vi "SelectOPCTags.AddItems.vi"(6 "VS Refs":T1[](array[typedef]) format="%.0x", 8 "error in (no error)":errorcluster, 9 "LUT":variant, 10 "Items":string[](array[string]), 11 "TreeControl in":refnum<vi>) -> (0 "error out":errorcluster)   [LabVIEW 2019, in "OPC UA Client Addon System Explorer.lvlib"]
uses:
  OPC UA Client Addon System Explorer.lvlib
  <vilib>/NI VeriStand/Custom Device API/Custom Device Item Ref.ctl
  Types/Tag.TreeSettings.ctl
  <vilib>/NI VeriStand/Custom Device API/Custom Device Channel.ctl
  <vilib>/NI VeriStand/Custom Device API/Custom Device Channel Type.ctl
  Addon Shared/Constants.vi
  <vilib>/NI VeriStand/Custom Device API/Set Item Property (U32).vi
  <vilib>/NI VeriStand/Custom Device API/Set Item Property (String).vi
  <vilib>/NI VeriStand/Custom Device API/Custom Device API.lvlib
  Addon Shared/OPC UA Client Addon Shared.lvlib
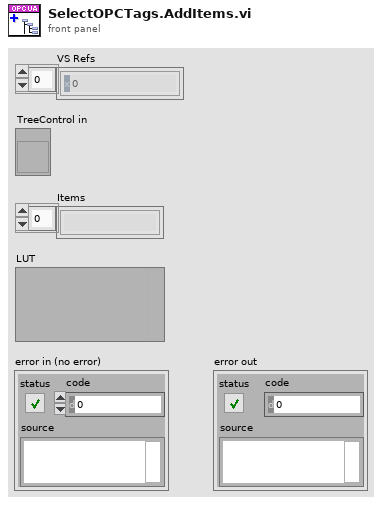
[diagram p1: front panel]
types:
  T1 = typedef "Custom Device API.lvlib/Custom Device Item Ref.ctl" = u64
  T2 = typedef "OPC UA Client Addon System Explorer.lvlib/Tag.TreeSettings.ctl" = cluster{"Settings":cluster{"name":string, "node type":enum32{"Other", "Folder", "Item/Property"}, "DataType":u32, "access":enum16{"Null", "Read", "Write", "Read&Write"}, "description":string}, "Array Size":i32}
  T3 = typedef "Custom Device API.lvlib/Custom Device Channel.ctl" = cluster{"Type":T4, "Units":string, "Default Value":dbl, "Faultable":bool, "Scalable":bool}
  T4 = typedef "Custom Device API.lvlib/Custom Device Channel Type.ctl" = enum16{"Input", "Output"}
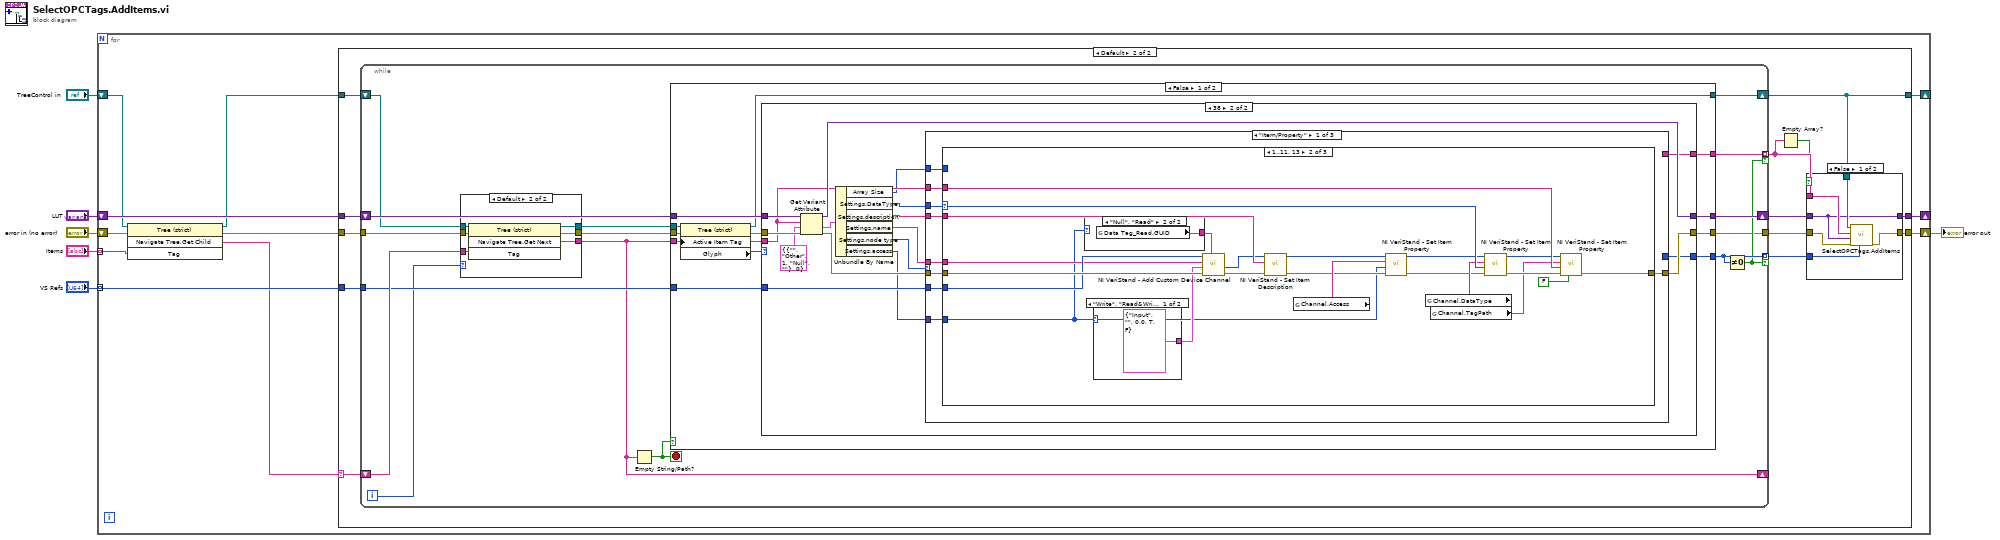
[diagram p0: block diagram]
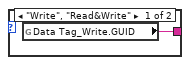
[diagram p7: hidden frame]
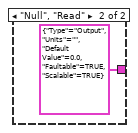
[diagram p8: hidden frame]
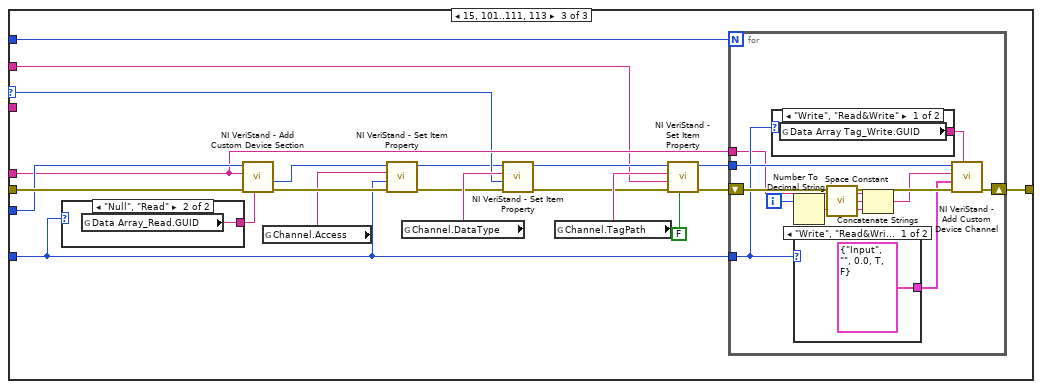
[diagram p9: hidden frame]
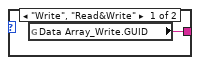
[diagram p10: hidden frame]
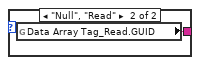
[diagram p11: hidden frame]
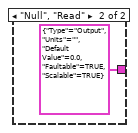
[diagram p12: hidden frame]
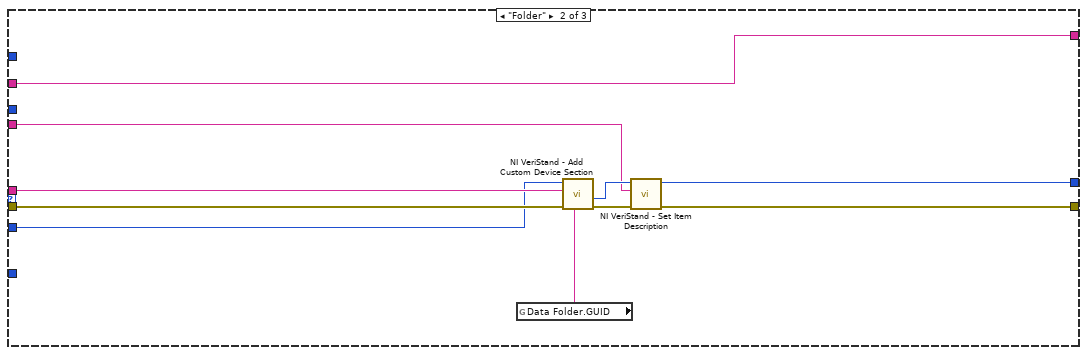
[diagram p13: hidden frame]
diagram:
  n1 = for {
    tunnel: "Items" -> [w8] mode=indexing
    tunnel: "VS Refs" -> [w17] mode=indexing
    shift-right: [w14] -> w1
    shift-left: "error in (no error)" -> [w12]
    shift-right: [w13] -> _
    shift-left: "LUT" -> [w16]
    shift-right: [w15] -> _
    shift-left: "TreeControl in" -> [w10]
    n2 = invoke class="Tree (strict)" method="Navigate Tree.Get Child"(reference=w10, error in=w12, "Tag"=w8) -> (reference out=w9:refnum<vi>, error out=w11:errorcluster, "Navigate Tree:Get Child"=w7:string)  [unwired: 1 in, 1 out]
    n3 = case shown="Default" w7 {
      selector: w7 -> [_ w21]
      tunnel: w17 -> [_ w33]
      tunnel: w16 -> [w19 w32]
      tunnel: [w20 w31] -> w15
      tunnel: [w18 w28] -> w14
      tunnel: [w19 w24] -> w13
      tunnel: w11 -> [w18 w23]
      tunnel: w9 -> [w20 w22]
      frame "" {
      }
      frame Default {
        n4 = while {
          tunnel: w23 -> [w56]
          shift-right: [w53] -> w30
          shift-left: w32 -> [w57]
          tunnel: [w51] -> w29 mode=indexing if=w49
          tunnel: [w50] -> w26 mode=indexing if=w49
          tunnel: w33 -> [w47]
          tunnel: [w46] -> w27
          shift-right: [w45] -> w31
          shift-left: w22 -> [w44]
          shift-right: [w43] -> _
          shift-left: w21 -> [w48]
          i -> [w42]
          stop <- w52 stop-if-true
          n5 = case shown="Default" w42 {
            tunnel: w56 -> [w59 w66]
            tunnel: [w58 w65] -> w55
            tunnel: [w59 w64] -> w54
            tunnel: w48 -> [w60 w63]
            tunnel: w44 -> [w58 w62]
            tunnel: [w60 w61] -> w43
            frame 0 {
            }
            frame Default {
              n6 = invoke class="Tree (strict)" method="Navigate Tree.Get Next"(reference=w62, error in=w66, "Tag"=w63) -> (reference out=w65:refnum<vi>, error out=w64:errorcluster, "Navigate Tree:Get Next Item"=w61:string)  [unwired: 1 in, 1 out]
            }
          }
          n7 = Empty String/Path?(string/path=w43) -> (empty?=w52:bool)
          n8 = case shown="False" w52 {
            tunnel: w57 -> [w78 w184]
            tunnel: w55 -> [w77 w183]
            tunnel: w54 -> [w76 w185]
            tunnel: w43 -> [w73 _]
            tunnel: [w72 w184] -> w53
            tunnel: [w71 w185] -> w46
            tunnel: [w70 _] -> w51
            tunnel: [w69 _] -> w50
            tunnel: w47 -> [w68 _]
            tunnel: [w67 w183] -> w45
            frame False {
              n9 = property class="Tree (strict)"(reference=w77, error in=w76, "Active Item Tag"=w73) -> (reference out=w67:refnum<vi>, error out=w75:errorcluster, "Glyph"=w74:i32)
              n10 = case shown="38" w74 {
                tunnel: w78 -> [w79 w97]
                tunnel: [w79 w96] -> w72
                tunnel: w75 -> [w80 w95]
                tunnel: w73 -> [_ w90]
                tunnel: [w80 w92] -> w71
                tunnel: [_ w91] -> w70
                tunnel: [_ w89] -> w69
                tunnel: w68 -> [_ w88]
                frame Default {
                }
                frame 38 {
                  n11 = Get Variant Attribute(Variant=w97, name=w90, default value (empty Variant)=T2 {"Settings"={"name"="", "node type"=enum."Other", "DataType"=1, "access"=enum."Null", "description"=""}, "Array Size"=0}, error in=w95) -> (duplicate Variant=w96:variant, value=w93:T2, error out=w94:errorcluster)  [unwired: 1 out]
                  n12 = Unbundle By Name(w93) -> ("Array Size"=w81:i32, "Settings.DataType"=w84:u32, "Settings.description"=w85:string, "Settings.name"=w87:string, "Settings.node type"=w86:enum32{"Other", "Folder", "Item/Property"}, "Settings.access"=w83:enum16{"Null", "Read", "Write", "Read&Write"})
                  n13 = case shown="\"Item/Property\"" w86 {
                    tunnel: w87 -> [w104 w181 _]
                    tunnel: w94 -> [w106 w180 w182]
                    tunnel: [_ w174 _] -> w91
                    tunnel: [w102 w176 w182] -> w92
                    tunnel: [_ w179 _] -> w89
                    tunnel: w90 -> [w101 w179 _]
                    tunnel: w88 -> [w105 w178 _]
                    tunnel: w85 -> [w103 w173 _]
                    tunnel: w84 -> [w99 _ _]
                    tunnel: w83 -> [w100 _ _]
                    tunnel: w81 -> [w98 _ _]
                    frame "Item/Property" {
                      n14 = case shown="1..11, 13" w99 {
                        selector: w99 -> [_ w123 w140]
                        tunnel: w106 -> [w107 w129 w153]
                        tunnel: w105 -> [_ w128 w152]
                        tunnel: w104 -> [_ w127 w151]
                        tunnel: w103 -> [_ w126 _]
                        tunnel: [w107 w125 w154] -> w102
                        tunnel: w101 -> [_ w124 w141]
                        tunnel: w100 -> [_ w108 w135]
                        tunnel: w98 -> [_ _ w150]
                        frame Default {
                        }
                        frame 1..11, 13 {
                          n15 = case shown="\"Null\", \"Read\"" w108 {
                            tunnel: [w130 w131] -> w114
                            frame "Write", "Read&Write" {
                              n16 = global read "Constants.vi" "Data Tag_Write.GUID"() -> (w130:string)
                            }
                            frame "Null", "Read" {
                              n17 = global read "Constants.vi" "Data Tag_Read.GUID"() -> (w131:string)
                            }
                          }
                          n18 = case shown="\"Write\", \"Read&Write\"" w108 {
                            tunnel: [T3 {"Type"=enum."Input", "Units"="", "Default Value"=0.0, "Faultable"=TRUE, "Scalable"=FALSE} ("Channel") T3 {"Type"=enum."Output", "Units"="", "Default Value"=0.0, "Faultable"=TRUE, "Scalable"=TRUE} ("Channel")] -> w118
                            frame "Write", "Read&Write" {
                            }
                            frame "Null", "Read" {
                            }
                          }
                          n19 = call <vilib>:"NI VeriStand - Add Custom Device Channel.vi"("GUID (Default Channel)"=w114, "error in (no error)"=w129, "Channel"=w118, "Channel Name"=w127, "Parent Ref in"=w128) -> ("error out"=w122:errorcluster, "Channel Ref"=w121:T1)  [unwired: 3 in, 2 out]
                          n20 = call <vilib>:"NI VeriStand - Set Item Description.vi"("error in (no error)"=w122, "Description"=w126, "Item Ref in"=w121) -> ("error out"=w112:errorcluster, "Item Ref out"=w110:T1)  [unwired: 6 in, 1 out]
                          n21 = global read "Constants.vi" "Channel.Access"() -> (w113:string)
                          n22 = call-poly <vilib>:"NI VeriStand - Set Item Property.vi"("error in (no error)"=w112, "Value"=w108, "Property Name"=w113, "Item Ref in"=w110) -> ("error out"=w111:errorcluster, "Item Ref out"=w109:T1)  [unwired: 5 in, 1 out]
                          n23 = global read "Constants.vi" "Channel.DataType"() -> (w117:string)
                          n24 = global read "Constants.vi" "Channel.TagPath"() -> (w116:string)
                          n25 = call-poly <vilib>:"NI VeriStand - Set Item Property.vi"("error in (no error)"=w111, "Value"=w123, "Property Name"=w117, "Item Ref in"=w109) -> ("error out"=w119:errorcluster, "Item Ref out"=w120:T1)  [unwired: 5 in, 1 out]
                          n26 = call-poly <vilib>:"NI VeriStand - Set Item Property.vi"("Binary String (T)"=FALSE, "error in (no error)"=w119, "Value"=w124, "Property Name"=w116, "Item Ref in"=w120) -> ("error out"=w125:errorcluster)  [unwired: 4 in, 2 out]
                        }
                        frame 15, 101..111, 113 {
                          n27 = case shown="\"Null\", \"Read\"" w135 {
                            tunnel: [w155 w156] -> w149
                            frame "Write", "Read&Write" {
                              n28 = global read "Constants.vi" "Data Array_Write.GUID"() -> (w155:string)
                            }
                            frame "Null", "Read" {
                              n29 = global read "Constants.vi" "Data Array_Read.GUID"() -> (w156:string)
                            }
                          }
                          n30 = call <vilib>:"NI VeriStand - Add Custom Device Section.vi"("GUID (Default Section)"=w149, "error in (no error)"=w153, "Section Name"=w151, "Parent Ref in"=w152) -> ("error out"=w139:errorcluster, "Section Ptr"=w137:T1)  [unwired: 4 in, 2 out]
                          n31 = global read "Constants.vi" "Channel.Access"() -> (w134:string)
                          n32 = call-poly <vilib>:"NI VeriStand - Set Item Property.vi"("error in (no error)"=w139, "Value"=w135, "Property Name"=w134, "Item Ref in"=w137) -> ("error out"=w138:errorcluster, "Item Ref out"=w136:T1)  [unwired: 5 in, 1 out]
                          n33 = global read "Constants.vi" "Channel.DataType"() -> (w146:string)
                          n34 = call-poly <vilib>:"NI VeriStand - Set Item Property.vi"("error in (no error)"=w138, "Value"=w140, "Property Name"=w146, "Item Ref in"=w136) -> ("error out"=w145:errorcluster, "Item Ref out"=w144:T1)  [unwired: 5 in, 1 out]
                          n35 = global read "Constants.vi" "Channel.TagPath"() -> (w147:string)
                          n36 = call-poly <vilib>:"NI VeriStand - Set Item Property.vi"("Binary String (T)"=FALSE, "error in (no error)"=w145, "Value"=w141, "Property Name"=w147, "Item Ref in"=w144) -> ("error out"=w142:errorcluster, "Item Ref out"=w143:T1)  [unwired: 4 in, 1 out]
                          n37 = for {
                            N: w150 -> [_]
                            tunnel: w143 -> [w166]
                            tunnel: w135 -> [w164]
                            shift-right: [w157] -> w154
                            shift-left: w142 -> [w167]
                            tunnel: w151 -> [w159]
                            i -> [w162]
                            n38 = case shown="\"Write\", \"Read&Write\"" w164 {
                              tunnel: [w168 w169] -> w163
                              frame "Write", "Read&Write" {
                                n39 = global read "Constants.vi" "Data Array Tag_Write.GUID"() -> (w168:string)
                              }
                              frame "Null", "Read" {
                                n40 = global read "Constants.vi" "Data Array Tag_Read.GUID"() -> (w169:string)
                              }
                            }
                            n41 = Number To Decimal String(number=w162) -> (decimal integer string=w161:string)  [unwired: 1 in]
                            n42 = case shown="\"Write\", \"Read&Write\"" w164 {
                              tunnel: [T3 {"Type"=enum."Input", "Units"="", "Default Value"=0.0, "Faultable"=TRUE, "Scalable"=FALSE} ("Channel") T3 {"Type"=enum."Output", "Units"="", "Default Value"=0.0, "Faultable"=TRUE, "Scalable"=TRUE} ("Channel")] -> w165
                              frame "Write", "Read&Write" {
                              }
                              frame "Null", "Read" {
                              }
                            }
                            n43 = call <vilib>:"Space Constant.vi"() -> ("String"=w158:string)
                            n44 = Concatenate Strings(w159, w158, w161) -> (w160:string)
                            n45 = call <vilib>:"NI VeriStand - Add Custom Device Channel.vi"("GUID (Default Channel)"=w163, "error in (no error)"=w167, "Channel"=w165, "Channel Name"=w160, "Parent Ref in"=w166) -> ("error out"=w157:errorcluster)  [unwired: 3 in, 3 out]
                          }
                        }
                      }
                    }
                    frame "Folder" {
                      n46 = global read "Constants.vi" "Data Folder.GUID"() -> (w172:string)
                      n47 = call <vilib>:"NI VeriStand - Add Custom Device Section.vi"("GUID (Default Section)"=w172, "error in (no error)"=w180, "Section Name"=w181, "Parent Ref in"=w178) -> ("error out"=w177:errorcluster, "Section Ptr"=w175:T1)  [unwired: 4 in, 2 out]
                      n48 = call <vilib>:"NI VeriStand - Set Item Description.vi"("error in (no error)"=w177, "Description"=w173, "Item Ref in"=w175) -> ("error out"=w176:errorcluster, "Item Ref out"=w174:T1)  [unwired: 6 in, 1 out]
                    }
                    frame "Other" {
                    }
                  }
                }
              }
            }
            frame True {
            }
          }
          n49 = Not Equal To 0?(x=w51) -> (x != 0?=w49:bool)
        }
        n50 = Empty Array?(array=w26) -> (empty?=w25:bool)
        n51 = case shown="False" w25 {
          tunnel: w31 -> [w39 _]
          tunnel: w26 -> [w38 _]
          tunnel: w30 -> [w34 w40]
          tunnel: w29 -> [w37 _]
          tunnel: [w36 w41] -> w28
          tunnel: w27 -> [w35 w41]
          tunnel: [w34 w40] -> w24
          frame False {
            n52 = call "SelectOPCTags.AddItems.vi"("VS Refs"=w37, "error in (no error)"=w35, "LUT"=w34, "Items"=w38, "TreeControl in"=w39) -> ("error out"=w36:errorcluster)  [unwired: 6 in]
          }
          frame True {
          }
        }
      }
    }
  }
  "error out" <- w1
